vi "Close Queues Command Based Example.vi"(8 "error in (no error)":errorcluster, 11 "FIFOs In":T1) -> (0 "error out":errorcluster)   [LabVIEW 2013]
uses:
  Command Based Example Queue Refs.ctl
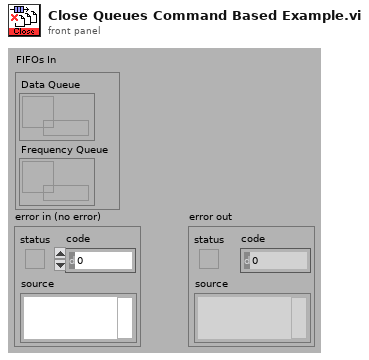
[diagram p1: front panel]
types:
  T1 = typedef "Command Based Example Queue Refs.ctl" = cluster{"Data Queue":refnum<queue>, "Frequency Queue":refnum<queue>}
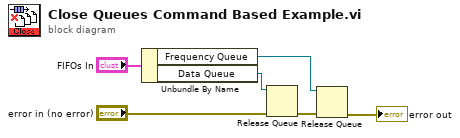
[diagram p0: block diagram]
diagram:
  n1 = Unbundle By Name("FIFOs In") -> ("Frequency Queue"=w3:refnum<queue>, "Data Queue"=w5:refnum<queue>)
  n2 = Release Queue(queue=w5, error in (no error)="error in (no error)") -> (error out=w4:errorcluster)  [unwired: 3 out]
  n3 = Release Queue(queue=w3, error in (no error)=w4) -> (error out=→"error out":errorcluster)  [unwired: 3 out]
